vi "Is Unset.vi"(4 "VolatusConfigElement in":refnum<class "VolatusConfigElement.lvclass">) -> (7 "Unset":bool)   [LabVIEW 2023, in "VolatusConfig.lvlib" / "VolatusConfigElement.lvclass"]
uses:
  VolatusConfigElement.lvclass
  VolatusConfigElement.lvclass/VolatusConfigElement.ctl
  lv-cdm/CDM-Config/Config Element/Config Element.lvclass
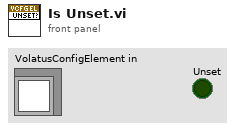
[diagram p1: front panel]
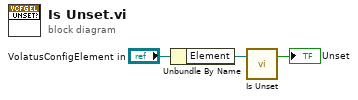
[diagram p0: block diagram]
diagram:
  n1 = Unbundle By Name("VolatusConfigElement in") -> ("Element"=w2:refnum<class "Config Element.lvclass">)
  n2 = call "Is Unset.vi"("Config Element in"=w2) -> ("Unset"=→"Unset":bool)  [unwired: 6 in]
